vi "Write Header Info.vi"(8 "error in (no error)":errorcluster, 10 "Header Info":u32, 11 "Node Ptr":T1 format="%.0x") -> (0 "error out":errorcluster, 3 "Node Ptr out":T1 format="%.0x")   [LabVIEW 2019, in "UDP-Custom-Device System Explorer.lvlib" / "Shared Packet Accessors.lvlib"]
uses:
  <vilib>/NI VeriStand/Custom Device API/Custom Device Item Ref.ctl
  Shared/Constants.vi
  <vilib>/NI VeriStand/Custom Device API/Set Item Property (U32).vi
  Shared Packet Accessors.lvlib
  <vilib>/NI VeriStand/Custom Device API/Custom Device API.lvlib
  Shared/UDP-Custom-Device Shared.lvlib
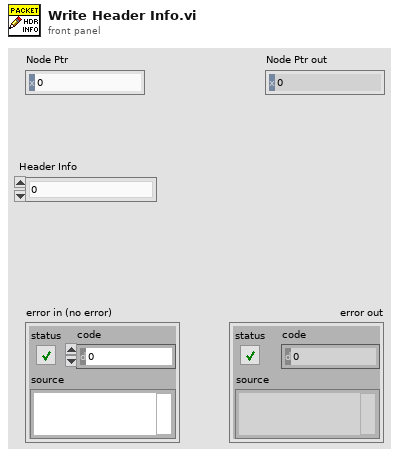
[diagram p1: front panel]
types:
  T1 = typedef "Custom Device API.lvlib/Custom Device Item Ref.ctl" = u64
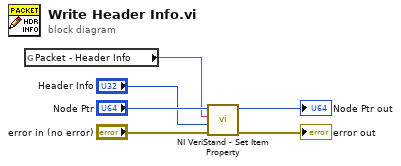
[diagram p0: block diagram]
diagram:
  n1 = global read "Constants.vi" "Packet - Header Info"() -> (w2:string)
  n2 = call-poly <vilib>:"NI VeriStand - Set Item Property.vi"("error in (no error)"="error in (no error)", "Value"="Header Info", "Property Name"=w2, "Item Ref in"="Node Ptr") -> ("error out"=→"error out":errorcluster, "Item Ref out"=→"Node Ptr out":T1)  [unwired: 5 in, 1 out]
